vi "Queue FGV.vi"(7 "Action":enum16{"Get", "Set"}(ring), 8 "error in":errorcluster, 11 "Command Queue":refnum<queue>) -> (0 "error out":errorcluster, 3 "Command Queue Out":refnum<queue>)   [LabVIEW 2011, in "Plugin Handler Command.lvclass"]
uses:
  Plugin Handler Command.lvclass
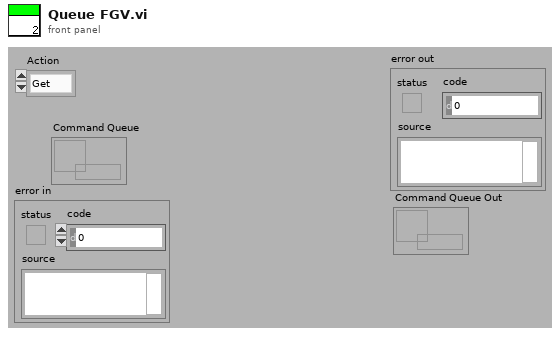
[diagram p1: front panel]
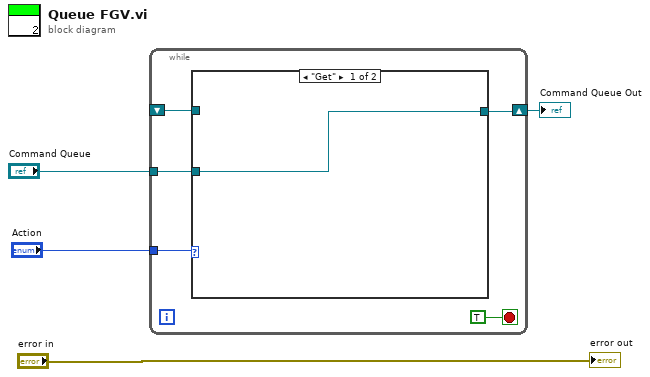
[diagram p0: block diagram]
diagram:
  n1 = while {
    tunnel: "Command Queue" -> [w8]
    tunnel: "Action" -> [w7]
    shift-right: [w6] -> w1
    shift-left: _ -> [w5]
    stop <- TRUE stop-if-true
    n2 = case shown="\"Get\"" w7 {
      tunnel: w8 -> [w10 _]
      tunnel: [w10 w11] -> w6
      tunnel: w5 -> [_ w11]
      frame "Get" {
      }
      frame "Set" {
      }
    }
  }
  "Command Queue Out" <- w1
  "error out" <- "error in"
